vi "vaj timing control.vi"(8 "J":dbl, 9 "A":dbl, 10 "V":dbl, 11 "D":dbl) -> (3 "Array":cluster{"Numeric":dbl, "Numeric":dbl}[](array[cluster]))   [LabVIEW 2019]
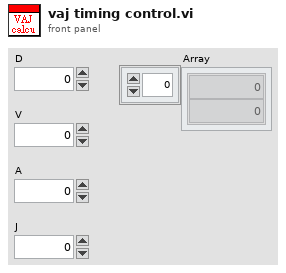
[diagram p1: front panel]
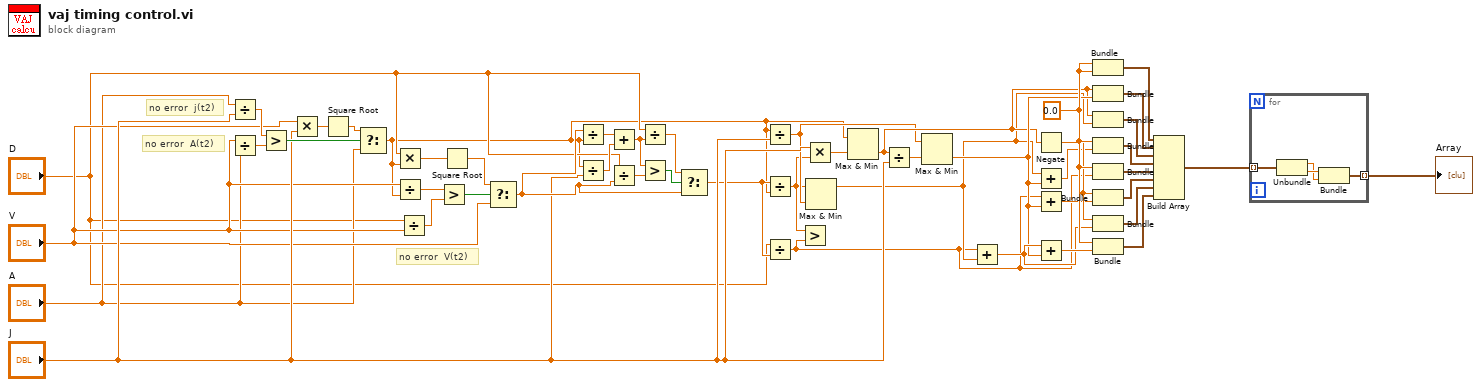
[diagram p0: block diagram]
diagram:
  w22 = 0.0
  # "no error  j(t2)"
  # "no error  A(t2)"
  # "no error  V(t2)"
  n1 = Divide(x="A", y="J") -> (x/y=w44:dbl)
  n2 = Divide(x="V", y="A") -> (x/y=w43:dbl)
  n3 = Greater?(x=w44, y=w43) -> (0:w46:bool)
  n4 = Multiply(x="V", y="J") -> (x*y=w38:dbl)
  n5 = Square Root(x=w38) -> (sqrt(x)=w47:dbl)
  n6 = Select(t=w47, s=w46, f="A") -> (s? t:f=w3:dbl)
  n7 = Multiply(x="D", y=w3) -> (x*y=w42:dbl)
  n8 = Divide(x="V", y=w3) -> (x/y=w39:dbl)
  n9 = Divide(x="D", y="V") -> (x/y=w45:dbl)
  n10 = Greater?(x=w39, y=w45) -> (0:w40:bool)
  n11 = Square Root(x=w42) -> (sqrt(x)=w41:dbl)
  n12 = Select(t=w41, s=w40, f="V") -> (s? t:f=w33:dbl)
  n13 = Divide(x=w33, y=w3) -> (x/y=w35:dbl)
  n14 = Divide(x=w3, y="J") -> (x/y=w36:dbl)
  n15 = Add(x=w35, y=w36) -> (x+y=w32:dbl)
  n16 = Divide(x="D", y=w33) -> (x/y=w37:dbl)
  n17 = Divide(x="D", y=w32) -> (x/y=w31:dbl)
  n18 = Greater?(x=w32, y=w37) -> (0:w34:bool)
  n19 = Select(t=w31, s=w34, f=w33) -> (s? t:f=w5:dbl)
  n20 = Divide(x=w3, y="J") -> (x/y=w11:dbl)
  n21 = Divide(x=w5, y=w3) -> (x/y=w9:dbl)
  n22 = Divide(x="D", y=w5) -> (x/y=w8:dbl)
  n23 = Greater?(x=w9, y=w8) -> ()  [unwired: 1 out]
  n24 = Multiply(x="J", y=w9) -> (x*y=w10:dbl)
  n25 = Max & Min(x=w9, y=w11) -> (max(x,y)=w12:dbl)  [unwired: 1 out]
  n26 = Max & Min(x=w3, y=w10) -> (min(x,y)=w14:dbl)  [unwired: 1 out]
  n27 = Divide(x=w14, y="J") -> (x/y=w13:dbl)
  n28 = Max & Min(x=w11, y=w13) -> (min(x,y)=w16:dbl)  [unwired: 1 out]
  n29 = Add(x=w8, y=w12) -> (x+y=w20:dbl)
  n30 = Negate(x=w14) -> (-x=w19:dbl)
  n31 = Add(x=w12, y=w16) -> (x+y=w17:dbl)
  n32 = Add(x=w8, y=w16) -> (x+y=w18:dbl)
  n33 = Add(x=w20, y=w16) -> (x+y=w21:dbl)
  n34 = Bundle(w22, w22) -> (w23:cluster{dbl, dbl})  [unwired: 1 in]
  n35 = Bundle(w14, w16) -> (w24:cluster{dbl, dbl})  [unwired: 1 in]
  n36 = Bundle(w14, w12) -> (w25:cluster{dbl, dbl})  [unwired: 1 in]
  n37 = Bundle(w22, w17) -> (w26:cluster{dbl, dbl})  [unwired: 1 in]
  n38 = Bundle(w22, w8) -> (w27:cluster{dbl, dbl})  [unwired: 1 in]
  n39 = Bundle(w19, w18) -> (w28:cluster{dbl, dbl})  [unwired: 1 in]
  n40 = Bundle(w19, w20) -> (w29:cluster{dbl, dbl})  [unwired: 1 in]
  n41 = Bundle(w22, w21) -> (w30:cluster{dbl, dbl})  [unwired: 1 in]
  n42 = Build Array(w23, w24, w25, w26, w27, w28, w29, w30) -> (w2:cluster{dbl, dbl}[])
  n43 = for {
    tunnel: w2 -> [w51] mode=indexing
    tunnel: [w48] -> w1 mode=indexing
    n44 = Unbundle(w51) -> (w49:dbl, w50:dbl)
    n45 = Bundle(w50, w49) -> (w48:cluster{dbl, dbl})  [unwired: 1 in]
  }
  "Array" <- w1
